vi "HFRR ADV v036.vi"() -> ()   [LabVIEW 2025] (continued)
                    tunnel: w3951 -> [_ _ _ _ _ _ _ _ _ _ _ _ _ _ _]
                    frame 0 {
                      "TITTLE" <- w3958
                    }
                    frame 1 {
                      "Sample ID" <- w3959
                    }
                    frame 2 {
                    }
                    frame 3 {
                    }
                    frame 4 {
                      "Test Date" <- w3960
                    }
                    frame 5 {
                      "Tested by" <- w3961
                    }
                    frame 6 {
                      n2894 = Fract/Exp String To Number(string=w3962) -> (number=→"Humidity before test 2":dbl)  [unwired: 3 in, 1 out]
                    }
                    frame 7 {
                      n2895 = Fract/Exp String To Number(string=w3964) -> (number=→"Temperature before test 2":dbl)  [unwired: 3 in, 1 out]
                    }
                    frame 8 {
                      n2896 = Fract/Exp String To Number(string=w3966) -> (number=→"Humidity after test 2":dbl)  [unwired: 3 in, 1 out]
                    }
                    frame 9 {
                      n2897 = Fract/Exp String To Number(string=w3968) -> (number=→"Temperature after test 2":dbl)  [unwired: 3 in, 1 out]
                    }
                    frame 10 {
                      n2898 = Fract/Exp String To Number(string=w3970) -> (number=→"MWSD 2":dbl)  [unwired: 3 in, 1 out]
                    }
                    frame 11 {
                      n2899 = Fract/Exp String To Number(string=w3972) -> (number=→"AVP 2":dbl)  [unwired: 3 in, 1 out]
                    }
                    frame 12 {
                      n2900 = Fract/Exp String To Number(string=w3974) -> (number=→"HCF 2":dbl)  [unwired: 3 in, 1 out]
                    }
                    frame 13 {
                      n2901 = Fract/Exp String To Number(string=w3976) -> (number=→"WS1.4 2":dbl)  [unwired: 3 in, 1 out]
                    }
                    frame 14, Default {
                    }
                  }
                }
              }
              frame #2 {
              }
            }
            n2902 = local write "OK Button 16"(FALSE ("OK Button 13")) -> ()
          }
        }
        n2903 = Index Array(array=w3621, index="Select Printer 3") -> (element=w3623:string)
        "Selected Printer" <- w3623
        n2904 = case shown="True" w3618 {
          frame False {
          }
          frame True {
            n2905 = flat-sequence {
              frame #0 {
              }
              frame #1 {
                n2906 = Wait (ms)(milliseconds to wait=u32 100) -> ()  [unwired: 1 out]
              }
              frame #2 {
                n2907 = local write "OK Button 16"(FALSE ("Print 3")) -> ()
              }
            }
          }
        }
        n2908 = case shown="True" "Print" {
          tunnel: w3623 -> [_ w3915]
          frame False {
          }
          frame True {
            (unwired) i16 6 ("width (-)")
            (unwired) "TESTED BY : "
            (unwired) "TESTED DATE :"
            (unwired) "SAMPLE ID : "
            (unwired) "SAMPLE DESIGN : "
            w3873 = "\r"
            w3890 = "\r"
            # "add image"
            n2909 = local read "Sample ID"() -> (w3863:string)
            n2910 = local read "Tested by"() -> (w3866:string)
            n2911 = local read "String 34"() -> (w3853:string)
            n2912 = local read "String 45"() -> (w3833:string)
            n2913 = local read "String 35"() -> (w3848:string)
            n2914 = local read "String 37"() -> (w3846:string)
            n2915 = local read "String 32"() -> (w3868:string)
            n2916 = local read "String 36"() -> (w3843:string)
            n2917 = local read "String 31"() -> (w3867:string)
            n2918 = local read "Test Date"() -> (w3864:string)
            n2919 = local read "String 33"() -> (w3869:string)
            n2920 = local read "String 38"() -> (w3839:string)
            n2921 = local read "String 39"() -> (w3836:string)
            n2922 = local write "Print"(FALSE ("Print FF")) -> ()
            n2923 = local read "S 39"() -> (w3851:string)
            n2924 = local read "S 38"() -> (w3858:string)
            n2925 = local read "Temperature before test 2"() -> (w3889:dbl)
            n2926 = local read "Temperature after test 2"() -> (w3879:dbl)
            n2927 = local read "Humidity before test 2"() -> (w3904:dbl)
            n2928 = local read "Humidity after test 2"() -> (w3888:dbl)
            n2929 = local read "MWSD 2"() -> (w3893:dbl)
            n2930 = local read "WS1.4 2"() -> (w3871:dbl)
            n2931 = Concatenate Strings("2)" ("string"), w3853) -> (w3854:string)
            n2932 = Concatenate Strings("3)" ("string"), w3851) -> (w3852:string)
            n2933 = Concatenate Strings("1)" ("string"), w3858) -> (w3857:string)
            n2934 = Concatenate Strings("4)" ("string"), w3848) -> (w3849:string)
            n2935 = Concatenate Strings("5)" ("string"), w3846) -> (w3845:string)
            n2936 = Concatenate Strings("6)" ("string"), w3843) -> (w3842:string)
            n2937 = Concatenate Strings("7)" ("string"), w3839) -> (w3840:string)
            n2938 = Concatenate Strings("8)" ("string"), w3836) -> (w3837:string)
            n2939 = local read "HCF 2"() -> (w3875:dbl)
            n2940 = local read "AVP 2"() -> (w3892:dbl)
            n2941 = local read "s.NO"() -> (w3834:string)
            n2942 = call <vilib>:"New Report.vi"("report type"=enum16{"Standard Report", "HTML"}."Standard Report") -> ("report out"=w3913:refnum<class "NI_report.lvclass">, "error out"=w3912:errorcluster)  [unwired: 13 in]
            n2943 = local read "TITTLE"() -> (w3865:string)
            n2944 = Concatenate Strings(w3890, w3833, w3834, w3890, w3868, w3863, w3890, w3867, w3864, w3890, w3869, w3866, w3890) -> (w3883:string)
            "test by" <- w3883
            n2945 = Number To Fractional String(number=w3889, width (-)=i16 6, precision (6)=i16 2) -> (F-format string=w3878:string)  [unwired: 1 in]
            n2946 = Number To Fractional String(number=w3888, width (-)=i16 6, precision (6)=i16 2) -> (F-format string=w3891:string)  [unwired: 1 in]
            n2947 = Number To Fractional String(number=w3904, width (-)=i16 6, precision (6)=i16 2) -> (F-format string=w3909:string)  [unwired: 1 in]
            n2948 = Number To Fractional String(number=w3893, width (-)=i16 6, precision (6)=i16 2) -> (F-format string=w3895:string)  [unwired: 1 in]
            n2949 = Number To Fractional String(number=w3879, width (-)=i16 6, precision (6)=i16 2) -> (F-format string=w3880:string)  [unwired: 1 in]
            n2950 = Number To Fractional String(number=w3892, width (-)=i16 6, precision (6)=i16 2) -> (F-format string=w3894:string)  [unwired: 1 in]
            n2951 = Number To Fractional String(number=w3875, width (-)=i16 6, precision (6)=i16 2) -> (F-format string=w3874:string)  [unwired: 1 in]
            n2952 = Number To Fractional String(number=w3871, precision (6)=i16 2) -> (F-format string=w3870:string)  [unwired: 2 in]
            n2953 = call-dynamic "Set Report Header Text.vi"("report in"=w3913, "center header text"=w3865, "error in (no error)"=w3912) -> ("report out"=w3884:refnum<class "NI_report.lvclass">, "error out"=w3885:errorcluster)  [unwired: 11 in]
            n2954 = Concatenate Strings(w3873, w3857, w3909, w3873, w3854, w3878, w3873, w3852, w3891, w3873, w3849, w3880, w3873, w3845, w3895, w3873, w3842, w3894, w3873, w3840, w3874, w3873, w3837, w3870) -> (w3861:string)
            "export 2" <- w3861
            n2955 = call-poly <vilib>:"Append Report Text.vi"("report in"=w3884, "text"=w3883, "error in (no error)"=w3885) -> ("report out"=w3887:refnum<class "NI_report.lvclass">, "error out"=w3886:errorcluster)  [unwired: 9 in, 2 out]
            n2956 = local read "test by"() -> (w3860:string)
            n2957 = local read "TITTLE"() -> (w3862:string)
            n2958 = call-poly <vilib>:"Append Report Text.vi"("report in"=w3887, "error in (no error)"=w3886) -> ("report out"=w3908:refnum<class "NI_report.lvclass">, "error out"=w3906:errorcluster)  [unwired: 10 in, 2 out]
            n2959 = Concatenate Strings(w3862, w3861, w3860) -> (→"output":string)
            n2960 = call-poly <vilib>:"Append Report Text.vi"("report in"=w3908, "text"=w3861, "error in (no error)"=w3906) -> ("report out"=w3907:refnum<class "NI_report.lvclass">, "error out"=w3905:errorcluster)  [unwired: 9 in, 2 out]
            n2961 = call-dynamic "Print Report.vi"("report in"=w3907, "printer name (default)"=w3915, "error in (no error)"=w3905) -> ("report out"=w3917:refnum<class "NI_report.lvclass">, "error out"=w3918:errorcluster)  [unwired: 11 in]
            n2962 = call-dynamic "Dispose Report.vi"("report in"=w3917, "error in (no error)"=w3918) -> ()  [unwired: 13 in, 1 out]
          }
        }
        n2963 = case shown="True" "Print 2" {
          frame False {
          }
          frame True {
            n2964 = flat-sequence {
              frame #0 {
                n2965 = local read "s.NO"() -> (→"s.NO 2":string)
                n2966 = Wait (ms)(milliseconds to wait=u32 20) -> ()  [unwired: 1 out]
                n2967 = local read "Sample ID  3"() -> (→"Sample ID  6":string)
                n2968 = local read "Sample ID  4"() -> (→"Sample ID  7":string)
                n2969 = local read "Sample ID"() -> (→"Sample ID  2":string)
                n2970 = local read "Tested by"() -> (→"Tested by 2":string)
                n2971 = local read "Test Date"() -> (→"Test Date 2":string)
                n2972 = local read "Humidity after test 3"() -> (→"Humidity after test 4":dbl)
                n2973 = local read "Ref A Test Date :"() -> (→"TITTLE 4":string)
                n2974 = local read "Temperature before test 3"() -> (w3740:dbl)
                n2975 = local read "Temperature before test 3"() -> (→"Temperature after test 5":dbl)
                n2976 = local read "Temperature after test 3"() -> (→"Temperature after test 4":dbl)
                n2977 = local read "Humidity before test 3"() -> (→"Humidity before test 4":dbl)
                n2978 = local write "Temperature before test 3"(w3740) -> ()
                n2979 = local read "image data"() -> (w3731:T16)
                n2980 = String To Path(string="C:\\LAB-IQ\\im\\Temp_resized.jpg") -> (path=w3732:path)
                "path 2" <- w3732
                n2981 = call <vilib>:"Write JPEG File.vi"("image data"=w3731, "path to JPEG file"=w3732) -> ()  [unwired: 8 in, 2 out]
                "Ref A Test Date :" <- "Ref A Test Date :"
                "Ref B Test Date :" <- "Ref B Test Date :"
                "Ref B Scar Value :" <- "Ref B Scar Value :"
                "Ref A Scar Value :" <- "Ref A Scar Value :"
              }
              frame #1 {
                (unwired) HTML_Report_Image_Alignment."MIDDLE" ("alignment (default)")
                w3768 = u16 0 items=["portrait", "landscape"] ("orientation (portrait)")
                (unwired) HTML_Report_Image_Alignment."ABSMIDDLE" ("alignment (default)")
                (unwired) "TESTED BY : "
                (unwired) "TESTED DATE :"
                (unwired) "SAMPLE ID : "
                (unwired) "SAMPLE DESIGN : "
                w3801 = "\r"
                # "add image"
                n2982 = Wait (ms)(milliseconds to wait=u32 20) -> ()  [unwired: 1 out]
                n2983 = local read "Sample ID  2"() -> (w3794:string)
                n2984 = local read "Wear Scar X"() -> (w3766:dbl)
                "Length ( microns ) 2" <- w3766
                n2985 = local read "Wear Scar Y"() -> (w3765:dbl)
                "Wear Scar Y ( microns ) :" <- w3765
                n2986 = local read "Test Date 2"() -> (w3795:string)
                n2987 = local read "Tested by 2"() -> (w3796:string)
                n2988 = local read "String 46"() -> (w3792:string)
                n2989 = local read "String 48"() -> (w3798:string)
                n2990 = local read "String 47"() -> (w3797:string)
                n2991 = local read "String 49"() -> (w3799:string)
                n2992 = local read "String 10"() -> (w3752:string)
                n2993 = local read "s.NO 2"() -> (w3793:string)
                n2994 = Add(x=w3766, y=w3765) -> (x+y=w3764:dbl)
                n2995 = call <vilib>:"New Report.vi"("report type"=enum16{"Standard Report", "HTML"}."HTML") -> ("report out"=w3772:refnum<class "NI_report.lvclass">, "error out"=w3770:errorcluster)  [unwired: 13 in]
                n2996 = Concatenate Strings(w3801, w3792, w3793, w3801, w3798, w3794, w3801, w3797, w3795, w3801, w3799, w3796, w3801) -> (→"test by 2":string)
                n2997 = Concatenate Strings("C:\\LAB-IQ\\Data\\" ("string"), w3752, ".jpg" ("string")) -> ()  [unwired: 1 out]
                n2998 = Divide(x=w3764, y=2.0) -> (x/y=→"Mean Wear ( microns) :":dbl)
                n2999 = call-dynamic "Set Report Orientation.vi"("report in"=w3772, "orientation (portrait)"=w3768, "error in (no error)"=w3770) -> ("report out"=w3771:refnum<class "NI_report.lvclass">, "error out"=w3769:errorcluster)  [unwired: 11 in]
                n3000 = for {
                  N: 5 -> [_]
                  tunnel: w3771 -> [w3822]
                  tunnel: [w3821] -> w3750
                  tunnel: w3769 -> [w3820]
                  tunnel: [w3819] -> w3749
                  n3001 = call-dynamic "Set Report Tab Width.vi"("report in"=w3822, "error in (no error)"=w3820) -> ("report out"=w3821:refnum<class "NI_report.lvclass">, "error out"=w3819:errorcluster)  [unwired: 12 in]
                }
                n3002 = local read "TITTLE"() -> (w3767:string)
                n3003 = call-dynamic "Set Report Header Text.vi"("report in"=w3750, "center header text"=w3767, "error in (no error)"=w3749) -> ("report out"=w3788:refnum<class "NI_report.lvclass">, "error out"=w3787:errorcluster)  [unwired: 11 in]
                n3004 = for {
                  N: 1 -> [_]
                  tunnel: [w3826] -> w3774
                  tunnel: [w3825] -> w3773
                  tunnel: w3788 -> [w3824]
                  tunnel: w3787 -> [w3823]
                  n3005 = call-dynamic "New Report Line.vi"("report in"=w3824, "error in (no error)"=w3823) -> ("report out"=w3826:refnum<class "NI_report.lvclass">, "error out"=w3825:errorcluster)  [unwired: 12 in]
                }
                n3006 = for {
                  N: 2 -> [_]
                  tunnel: [w3818] -> w3780
                  tunnel: [w3817] -> w3779
                  tunnel: w3774 -> [w3816]
                  tunnel: w3773 -> [w3815]
                  n3007 = call-dynamic "New Report Line.vi"("report in"=w3816, "error in (no error)"=w3815) -> ("report out"=w3818:refnum<class "NI_report.lvclass">, "error out"=w3817:errorcluster)  [unwired: 12 in]
                }
                n3008 = for {
                  N: 25 -> [_]
                  tunnel: w3780 -> [w3814]
                  tunnel: w3779 -> [w3812]
                  tunnel: [w3813] -> w3783
                  tunnel: [w3811] -> w3782
                  n3009 = call-dynamic "Set Report Tab Width.vi"("report in"=w3814, "error in (no error)"=w3812) -> ("report out"=w3813:refnum<class "NI_report.lvclass">, "error out"=w3811:errorcluster)  [unwired: 12 in]
                }
                n3010 = control-ref of="Tab Control 9"() -> (w3778:refnum<vi>)
                n3011 = call-dynamic "Append Control Image to Report.vi"("report in"=w3783, "alignment (default)"=HTML_Report_Image_Alignment."ABSMIDDLE", "ctrl reference"=w3778, "error in (no error)"=w3782) -> ("report out"=w3777:refnum<class "NI_report.lvclass">, "error out"=w3776:errorcluster)  [unwired: 8 in, 2 out]
                n3012 = for {
                  N: 3 -> [_]
                  tunnel: [w3810] -> w3761
                  tunnel: [w3809] -> w3760
                  tunnel: w3777 -> [w3808]
                  tunnel: w3776 -> [w3807]
                  n3013 = call-dynamic "New Report Line.vi"("report in"=w3808, "error in (no error)"=w3807) -> ("report out"=w3810:refnum<class "NI_report.lvclass">, "error out"=w3809:errorcluster)  [unwired: 12 in]
                }
                n3014 = for {
                  N: 100 -> [_]
                  tunnel: w3761 -> [w3806]
                  tunnel: w3760 -> [w3804]
                  tunnel: [w3805] -> w3757
                  tunnel: [w3803] -> w3755
                  n3015 = call-dynamic "Set Report Tab Width.vi"("report in"=w3806, "error in (no error)"=w3804) -> ("report out"=w3805:refnum<class "NI_report.lvclass">, "error out"=w3803:errorcluster)  [unwired: 12 in]
                }
                n3016 = String To Path(string="C:\\LAB-IQ\\im\\Temp_resized.jpg") -> (path=w3747:path)
                n3017 = call-poly <vilib>:"Append Image to Report.vi"("report in"=w3757, "path or URL of image"=w3747, "error in (no error)"=w3755) -> ("report out"=w3756:refnum<class "NI_report.lvclass">, "error out"=w3754:errorcluster)  [unwired: 9 in, 2 out]
                n3018 = call-poly <vilib>:"Open HTML Report in Browser.vi"("report in"=w3756, "error in (no error)"=w3754) -> ("report out"=w3791:refnum<class "NI_report.lvclass">, "error out"=w3790:errorcluster)  [unwired: 11 in, 1 out]
                n3019 = call-dynamic "Dispose Report.vi"("report in"=w3791, "error in (no error)"=w3790) -> ()  [unwired: 13 in, 1 out]
              }
              frame #2 {
              }
              frame #3 {
                n3020 = disable-structure shown="Disabled" {
                  frame Disabled {
                    n3021 = local read "String 10"() -> (w3831:string)
                    n3022 = Concatenate Strings("C:\\LAB-IQ-NXT\\Data\\" ("string"), w3831, ".jpg" ("string")) -> (w3829:string)
                    n3023 = String To Path(string=w3829) -> (path=w3828:path)
                    n3024 = Delete(path (use dialog)=w3828) -> ()  [unwired: 4 in, 3 out]
                  }
                  frame Enabled {
                  }
                }
                n3025 = local write "Print 2"(FALSE ("Print")) -> ()
              }
            }
          }
        }
      }
    }
    n3026 = Wait (ms)(milliseconds to wait=u32 50) -> ()  [unwired: 1 out]
    n3027 = Wait (ms)(milliseconds to wait=u32 50) -> ()  [unwired: 1 out]
    n3028 = local read "Quit"() -> (w2175:bool)
  }
  n3029 = VISA Close(VISA resource name=w41, error in (no error)=w40) -> ()  [unwired: 1 out]
  n3030 = while {
    stop <- w3982 stop-if-true
    n3031 = local read "Auto Start Test"() -> (w3980:bool)
    n3032 = local read "RUN"() -> (w3979:bool)
    n3033 = Wait (ms)(milliseconds to wait=u32 1000) -> ()  [unwired: 1 out]
    n3034 = Or(x=w3979, y=w3980) -> (x .or. y?=w3978:bool)
    n3035 = case shown="True" w3978 {
      frame False {
      }
      frame True {
        n3036 = local read "LVDT STROKE Actual"() -> (w3983:dbl)
        n3037 = In Range and Coerce(upper limit=1.2, x=w3983, lower limit=0.6) -> (In Range?=w3986:bool)  [unwired: 1 out]
        n3038 = call-poly <vilib>:"Random Number (Range).vi"("lower bound (0)"=0.998 ("upper bound (100)"), "upper bound (100)"=1.003) -> ("number"=w3984:dbl)  [unwired: 9 in]
        n3039 = case shown="True" w3986 {
          tunnel: [w3991 w3992] -> w3985
          tunnel: w3984 -> [_ w3992]
          tunnel: w3983 -> [w3991 _]
          frame False {
          }
          frame True {
          }
        }
        "LVDT STROKE DISPLAY" <- w3985
      }
    }
    n3040 = local read "Quit"() -> (w3982:bool)
  }
  n3041 = while {
    tunnel: [w4009] -> w49
    shift-right: [w4002] -> _
    shift-left: 0.0 -> [w4005]
    shift-right: [w4001] -> _
    shift-left: 0.0 -> [w4004]
    shift-right: [w4000] -> _
    shift-left: 100.0 ("vc_cmd") -> [w4003]
    stop <- w4009 stop-if-true
    # "PID LOGIC"
    n3042 = local read "run test Calibration"() -> (w3997:bool)
    n3043 = local read "RUN"() -> (w4007:bool)
    n3044 = local read "Auto Start Temp"() -> (w3998:bool)
    n3045 = local read "Auto Start Test"() -> (w4006:bool)
    n3046 = local read "START TEMP"() -> (w3996:bool)
    n3047 = And(x=w3998, y=w4006) -> (x .and. y?=w3999:bool)
    n3048 = Or(x=w4007, y=w3999) -> (x .or. y?=w4008:bool)
    n3049 = And(x=w4008, y=w3996) -> (x .and. y?=w3995:bool)
    n3050 = And(x=w3997, y=w3996) -> (x .and. y?=w3994:bool)
    n3051 = Or(x=w3994, y=w3995) -> (x .or. y?=w3993:bool)
    n3052 = Wait (ms)(milliseconds to wait="milliseconds to wait") -> ()  [unwired: 1 out]
    n3053 = case shown="True" w3993 {
      tunnel: [400.0 ("out_vc_cmd") w4028] -> w4000
      tunnel: [w4012 w4030] -> w4001
      tunnel: [w4012 w4029] -> w4002
      tunnel: w4005 -> [_ w4019]
      tunnel: w4004 -> [_ w4018]
      tunnel: w4003 -> [_ w4017]
      tunnel: w3997 -> [_ w4013]
      frame False {
        w4012 = 0.0 ("error_out")
      }
      frame True {
        n3054 = case shown="True" w4013 {
          tunnel: [w4037 1.0] -> w4015
          frame False {
            n3055 = local read "Set Strk"() -> (w4036:dbl)
            n3056 = Add(x=w4036, y="Add up Stroke") -> (x+y=w4037:dbl)
          }
          frame True {
          }
        }
        n3057 = local read "LVDT STROKE"() -> (w4014:dbl)
        n3058 = formula code="// Zero-Hardcode Explicit Positional-Form PID Engine\n// Inputs: target_stroke, measured_stroke, dt, prev_error, integral_accumulator_in, prev_vc_cmd\n//         kp, ki, kd, max_step_change, max_amplitude, min_amplitude, startup_cmd\n// Outputs: vc_cmd, error_out, out_error, integral_accumulator_out, out_vc_cmd\n\n// 1. Calculate Tracking Error\nfloat current_error = target_stroke - measured_stroke;\nerror_out = current_error;\n\n// 2. Compute Proportional Term\nfloat p_term = kp * current_error;\n\n// 3. Compute Derivative Term\nfloat d_term = 0.0;\nif (dt > 0.0) {\n    d_term = kd * ((current_error - prev_error) / dt);\n}\n\n// 4. Update and Accumulate Integral Term\nfloat current_integral = integral_accumulator_in + (current_error * dt);\nfloat i_term = ki * current_integral;\n\n// 5. Calculate Ideal Target Command (Anchored by startup baseline)\nfloat ideal_command = startup_cmd + p_term + i_term + d_term;\n\n// 6. Apply Loop Rate Limiting FIRST \n// (Forces the command to climb gradually from prev_vc_cmd instead of jumping straight to max)\nfloat raw_adjustment = ideal_command - prev_vc_cmd;\n\nif (raw_adjustment > max_step_change) {\n    raw_adjustment = max_step_change;\n} else if (raw_adjustment < -max_step_change) {\n    raw_adjustment = -max_step_change;\n}\n\nfloat next_vc_cmd = prev_vc_cmd + raw_adjustment;\n\n// 7. Anti-Windup Protection & Final Output Safety Safeguard Clamping\n// (Back-calculating based on what we are ACTUALLY outputting)\nif (next_vc_cmd > max_amplitude) {\n    float excess = next_vc_cmd - max_amplitude;\n    if (ki > 0.0) {\n        current_integral -= excess / ki;\n    }\n    next_vc_cmd = max_amplitude;\n} else if (next_vc_cmd < min_amplitude) {\n    float excess = next_vc_cmd - min_amplitude;\n    if (ki > 0.0) {\n        current_integral -= excess / ki;\n    }\n    next_vc_cmd = min_amplitude;\n}\n\n// 8. Map to Shift Registers for memory persistence\nvc_cmd = next_vc_cmd;\nout_error = current_error;                   \nintegral_accumulator_out = current_integral;  \nout_vc_cmd = next_vc_cmd;"("target_stroke"=w4015, "measured_stroke"=w4014, "dt"="dt", "integral_accumulator_in"=w4018, "prev_error"=w4019, "prev_vc_cmd"=w4017, "kp"="kp", "ki"="ki", "kd"="kd", "max_step_change"="max_step_change", "max_amplitude"="max_amplitude", "min_amplitude"="min_amplitude", "startup_cmd"="startup_cmd") -> ("vc_cmd"=w4034:dbl, "out_error"=w4029:dbl, "integral_accumulator_out"=w4030:dbl, "out_vc_cmd"=w4028:dbl)  [unwired: 1 out]
        "output Vpp" <- w4034
        n3059 = Number To Fractional String(number=w4034, precision (6)=i16 1) -> (F-format string=w4032:string)  [unwired: 2 in]
        n3060 = Concatenate Strings("DAC;" ("string"), w4032) -> (w4016:string)
        n3061 = local write "Due Write"(w4016) -> ()
        "prev_error" <- w4019
        "integral_accumulator_in" <- w4018
        "prev_vc_cmd" <- w4017
      }
    }
    n3062 = local read "Quit"() -> (w4009:bool)
  }
  n3063 = Or(x=w45, y=w44) -> (x .or. y?=w46:bool)
  n3064 = Or(x=w42, y=w46) -> (x .or. y?=w51:bool)
  n3065 = control-ref of="new picture"() -> ()  [unwired: 1 out]
  n3066 = Or(x=w54, y=w51) -> (x .or. y?=w48:bool)
  n3067 = Or(x=w48, y=w49) -> (x .or. y?=w43:bool)
  n3068 = while {
    tunnel: [w4039] -> w53
    i -> [w4046]
    stop <- w4039 stop-if-true
    n3069 = local read "Quit"() -> (w4039:bool)
    n3070 = Equal To 0?(x=w4046) -> (x = 0?=w4044:bool)
    n3071 = call "Elapsed Time3"("Time Target (s)"=45.0, "Auto Reset"=TRUE) -> ("Time has Elapsed"=w4043:bool)  [unwired: 10 in, 7 out]
    n3072 = Wait (ms)(milliseconds to wait=u32 50) -> ()  [unwired: 1 out]
    n3073 = Or(x=w4043, y=w4044) -> (x .or. y?=w4045:bool)
    n3074 = case shown="True" w4045 {
      frame False {
      }
      frame True {
        n3075 = call <vilib>:"System Exec.vi"("run minimized? (F)"=TRUE, "error in (no error)"="error in (no error)", "command line"="powercfg.exe -change -monitor-timeout-ac 0") -> ("error out"=w4057:errorcluster)  [unwired: 5 in, 3 out]
        n3076 = call <vilib>:"System Exec.vi"("run minimized? (F)"=TRUE, "error in (no error)"=w4057, "command line"="powercfg.exe -change -disk-timeout-ac 0") -> ("error out"=w4056:errorcluster)  [unwired: 5 in, 3 out]
        n3077 = call <vilib>:"System Exec.vi"("run minimized? (F)"=TRUE, "error in (no error)"=w4056, "command line"="powercfg.exe -change -standby-timeout-ac 0") -> ("error out"=w4055:errorcluster)  [unwired: 5 in, 3 out]
        n3078 = call <vilib>:"System Exec.vi"("run minimized? (F)"=TRUE, "error in (no error)"=w4055, "command line"="powercfg.exe -change -hibernate-timeout-ac 0") -> ("error out"=w4054:errorcluster)  [unwired: 5 in, 3 out]
        n3079 = call <vilib>:"Simple Error Handler.vi"("error in (no error)"=w4054) -> ("error out"=w4060:errorcluster)  [unwired: 4 in, 4 out]
        n3080 = call <vilib>:"Clear Errors.vi"("error in (no error)"=w4060) -> ("error out"=→"error out":errorcluster)  [unwired: 5 in, 1 out]
      }
    }
  }
  n3081 = Compound Arithmetic op=OR(w56, w43, w53) -> (w55:bool)
  n3082 = flat-sequence {
    tunnel: w55 -> [_]
    tunnel: [w4062] -> w25
    tunnel: w25 -> [_]
    frame #0 {
      n3083 = call "CLOSE CONNECTION.vi"() -> ("error out"=w4062:errorcluster)  [unwired: 11 in]
    }
    frame #1 {
      n3084 = Quit LabVIEW(quit? (T)=TRUE) -> ()
      n3085 = local write "Quit"(FALSE ("EXIT")) -> ()
    }
  }
  n3086 = property on="Heater Button" class="Bool (strict)"("Visible"=TRUE) -> ()  [unwired: 2 in, 2 out]
  n3087 = while {
    tunnel: [w4069] -> _
    i -> [w4069]
    stop <- w4065 stop-if-true
    # "Langauage selection"
    n3088 = Equal?(x="Lan flag", y=22.0) -> ()  [unwired: 1 out]
    n3089 = disable-structure shown="Disabled" {
      frame Disabled {
        n3090 = stacked-sequence {
          frame #0 {
            n3091 = case shown="\"Russian\"" "Language Selection" {
              tunnel: [0 1] -> w4071
              frame "English", Default {
              }
              frame "Russian" {
              }
            }
            n3092 = for {
              N: 130 -> [_]
              tunnel: "Table" -> [w4080]
              tunnel: w4071 -> [w4079]
              i -> [w4078]
              n3093 = Index Array(array=w4080, index (row)=w4078, index (col)=w4079) -> (element=w4077:string)
              n3094 = case shown="1" w4078 {
                tunnel: w4077 -> [w4081 w4082 _ w4083 w4084 w4085 w4086 w4087 w4088 w4089 w4090 w4091 w4092 w4093 w4094 w4095 w4096 w4097 w4098 w4099 w4100 w4101 w4102 w4103 w4104 w4105 w4106 w4107 w4108 _ _ w4109 w4110 w4111 w4112 w4113 w4114 w4123 w4130 w4137 w4144 w4148 w4151 w4154 w4156 w4158 w4159 w4160 w4161 w4162 w4163 w4164 w4165 w4166 w4167 w4168 w4169 w4170 w4171 w4172 w4173 w4174 w4175 w4176 w4177 w4178 w4179 w4180 w4181 w4182 w4183 w4184 w4185 w4186 w4187 w4188 w4189 w4190 w4191 w4192 w4193 w4194 w4195 w4196 w4197 w4198 w4199 w4200 w4201 w4202 w4203 w4204 w4205 w4206 w4207 w4208 w4209 w4210 w4211 w4212 w4213 w4214 w4215 w4216 w4217 _ w4218 w4219 w4220 w4221 w4222 w4223 w4224 w4225 w4226 w4227 w4228 w4229 w4230 _ w4231 w4232 w4233 w4234 w4235 w4236 _]
                frame 0 {
                  n3095 = local write "S"(w4081) -> ()
                }
                frame 1 {
                  n3096 = local write "S 2"(w4082) -> ()
                }
                frame 2 {
                }
                frame 3 {
                  n3097 = local write "S 4"(w4083) -> ()
                }
                frame 4 {
                  n3098 = property on="FILE" class="Str"("Caption.Text"=w4084) -> ()  [unwired: 2 in, 2 out]
                }
                frame 5 {
                  n3099 = property on="Fuel Discription :" class="Str"("Caption.Text"=w4085) -> ()  [unwired: 2 in, 2 out]
                }
                frame 6 {
                  n3100 = property on="Remarks :" class="Str"("Caption.Text"=w4086) -> ()  [unwired: 2 in, 2 out]
                }
                frame 7 {
                  n3101 = property on="Save & Continue" class="Bool (strict)"("Boolean Text.Text"=w4087) -> ()  [unwired: 2 in, 2 out]
                }
                frame 8 {
                }
                frame 9 {
                  n3102 = property on="Set Hz" class="DigNum (strict)"("Caption.Text"=w4089) -> ()  [unwired: 2 in, 2 out]
                }
                frame 10 {
                }
                frame 11 {
                  n3103 = property on="NORMAL LOAD" class="DigNum (strict)"("Caption.Text"=w4091) -> ()  [unwired: 2 in, 2 out]
                }
                frame 12 {
                }
                frame 13 {
                  n3104 = property on="Set Temp" class="DigNum (strict)"("Caption.Text"=w4093) -> ()  [unwired: 2 in, 2 out]
                }
                frame 14 {
                  n3105 = local write "S 15"(w4094) -> ()
                }
                frame 15 {
                  n3106 = property on="Set Rh" class="DigNum (strict)"("Caption.Text"=w4095) -> ()  [unwired: 2 in, 2 out]
                }
                frame 16 {
                }
                frame 17 {
                  n3107 = local write "S 18"(w4097) -> ()
                }
                frame 18 {
                  "String 17" <- w4098
                }
                frame 19 {
                  n3108 = property on="test time" class="DigNum (strict)"("Caption.Text"=w4099) -> ()  [unwired: 2 in, 2 out]
                }
                frame 20 {
                  "String 18" <- w4100
                  "String 22" <- w4100
                }
                frame 21 {
                  n3109 = property on="Elapsed time" class="DigNum (strict)"("Caption.Text"=w4101) -> ()  [unwired: 2 in, 2 out]
                }
                frame 22 {
                  n3110 = property on="Samplingtime 2" class="DigNum (strict)"("Caption.Text"=w4102) -> ()  [unwired: 2 in, 2 out]
                }
                frame 23 {
                  "String 21" <- w4103
                }
                frame 24 {
                  n3111 = property on="Countdown" class="DigNum (strict)"("Caption.Text"=w4104) -> ()  [unwired: 2 in, 2 out]
                }
                frame 25 {
                  n3112 = property on="Countdown 2" class="DigNum (strict)"("Caption.Text"=w4105) -> ()  [unwired: 2 in, 2 out]
                }
                frame 26 {
                  n3113 = property on="Engage" class="Bool (strict)"("Boolean Text.Text"=w4106) -> ()  [unwired: 2 in, 2 out]
                }
                frame 27 {
                  n3114 = property on="Boolean  4" class="Bool (strict)"("Boolean Text.Text"=w4107) -> ()  [unwired: 2 in, 2 out]
                }
                frame 28 {
                  n3115 = property on="Test \nStatus" class="Bool (strict)"("Boolean Text.Text"=w4108) -> ()  [unwired: 2 in, 2 out]
                }
                frame 29 {
                }
                frame 30 {
                }
                frame 31 {
                }
                frame 32 {
                  n3116 = property on="RSTCOF" class="Bool"("Boolean Text.Text"=w4110) -> ()  [unwired: 2 in, 2 out]
                  n3117 = property on="RST FF" class="Bool"("Boolean Text.Text"=w4110) -> ()  [unwired: 2 in, 2 out]
                  n3118 = property on="RST TEMP" class="Bool"("Boolean Text.Text"=w4110) -> ()  [unwired: 2 in, 2 out]
                  n3119 = property on="RSTV1 3" class="Bool"("Boolean Text.Text"=w4110) -> ()  [unwired: 2 in, 2 out]
                  n3120 = property on="rstv2" class="Bool"("Boolean Text.Text"=w4110) -> ()  [unwired: 2 in, 2 out]
                  n3121 = property on="RSTV1 2" class="Bool"("Boolean Text.Text"=w4110) -> ()  [unwired: 2 in, 2 out]
                  n3122 = property on="RST CP" class="Bool"("Boolean Text.Text"=w4110) -> ()  [unwired: 2 in, 2 out]
                }
                frame 33 {
                  "S 61" <- w4111
                }
                frame 34 {
                  "String 23" <- w4112
                }
                frame 35 {
                  n3123 = property on="Rh Before" class="DigNum (strict)"("Caption.Text"=w4113) -> ()  [unwired: 2 in, 2 out]
                }
                frame 36 {
                  n3124 = Match Pattern(string=w4114, regular expression=",") -> (before substring=→"bs":string, after substring=→"as":string)  [unwired: 1 in, 2 out]
                  n3125 = property on="Rh After" class="DigNum (strict)"("Caption.Text"=w4114) -> ()  [unwired: 2 in, 2 out]
                }
                frame 37 {
                  n3126 = Match Pattern(string=w4123, regular expression=",") -> (before substring=w4122:string, after substring=w4121:string)  [unwired: 1 in, 2 out]
                  "bs" <- w4122
                  "as" <- w4121
                  n3127 = Concatenate Strings(w4122, w4121) -> (w4118:string)
                  n3128 = property on="Humidity before test 2" class="DigNum (strict)"("Caption.Text"=w4118) -> ()  [unwired: 2 in, 2 out]
                  n3129 = Concatenate Strings(w4118, "=" ("string")) -> (w4119:string)
                  n3130 = local write "S 38"(w4119) -> ()
                }
                frame 38 {
                  n3131 = Match Pattern(string=w4130, regular expression=",") -> (before substring=w4129:string, after substring=w4128:string)  [unwired: 1 in, 2 out]
                  "bs" <- w4129
                  "as" <- w4128
                  n3132 = Concatenate Strings(w4129, w4128) -> (w4125:string)
                  n3133 = property on="Humidity after test 2" class="DigNum (strict)"("Caption.Text"=w4125) -> ()  [unwired: 2 in, 2 out]
                  n3134 = Concatenate Strings(w4125, "=" ("string")) -> (w4127:string)
                  n3135 = local write "S 39"(w4127) -> ()
                }
                frame 39 {
                  n3136 = Match Pattern(string=w4137, regular expression=",") -> (before substring=w4136:string, after substring=w4135:string)  [unwired: 1 in, 2 out]
                  "bs" <- w4136
                  "as" <- w4135
                  n3137 = Concatenate Strings(w4136, w4135) -> (w4132:string)
                  n3138 = property on="Temperature before test 2" class="DigNum (strict)"("Caption.Text"=w4132) -> ()  [unwired: 2 in, 2 out]
                  n3139 = Concatenate Strings(w4132, "=" ("string")) -> (→"String 34":string)
                }
                frame 40 {
                  n3140 = Match Pattern(string=w4144, regular expression=",") -> (before substring=w4143:string, after substring=w4142:string)  [unwired: 1 in, 2 out]
                  "bs" <- w4143
                  "as" <- w4142
                  n3141 = Concatenate Strings(w4143, w4142) -> (w4139:string)
                  n3142 = property on="Temperature after test 2" class="DigNum (strict)"("Caption.Text"=w4139) -> ()  [unwired: 2 in, 2 out]
                  n3143 = Concatenate Strings(w4139, "=" ("string")) -> (→"String 35":string)
                  n3144 = property on="Temperature after test" class="DigNum (strict)"("Caption.Text"=w4139) -> ()  [unwired: 2 in, 2 out]
                }
                frame 41 {
                  n3145 = property on="AVP 2" class="DigNum (strict)"("Caption.Text"=w4148) -> ()  [unwired: 2 in, 2 out]
                  n3146 = Concatenate Strings(w4148, "=" ("string")) -> (→"String 36":string)
                }
                frame 42 {
                  n3147 = property on="MWSD 2" class="DigNum (strict)"("Caption.Text"=w4151) -> ()  [unwired: 2 in, 2 out]
                  n3148 = Concatenate Strings(w4151, "=" ("string")) -> (→"String 37":string)
                }
                frame 43 {
                  n3149 = property on="HCF 2" class="DigNum (strict)"("Caption.Text"=w4154) -> ()  [unwired: 2 in, 2 out]
                  n3150 = Concatenate Strings(w4154, "=" ("string")) -> (→"String 38":string)
                }
                frame 44 {
                  n3151 = Concatenate Strings(w4156, "=" ("string")) -> (→"String 39":string)
                  n3152 = property on="WS1.4 2" class="DigNum (strict)"("Caption.Text"=w4156) -> ()  [unwired: 2 in, 2 out]
                }
                frame 45 {
                }
                frame 46 {
                  n3153 = local write "S 47"(w4159) -> ()
                }
                frame 47 {
                  n3154 = local write "S 48"(w4160) -> ()
                }
                frame 48 {
                  n3155 = local write "S 49"(w4161) -> ()
                }
                frame 49 {
                  n3156 = local write "S 50"(w4162) -> ()
                }
                frame 50 {
                  n3157 = local write "S 51"(w4163) -> ()
                }
                frame 51 {
                  n3158 = local write "S 52"(w4164) -> ()
                }
                frame 52 {
                  n3159 = local write "S 53"(w4165) -> ()
                }
                frame 53 {
                  n3160 = local write "S 54"(w4166) -> ()
                }
                frame 54 {
                  n3161 = local write "S 55"(w4167) -> ()
                }
                frame 55 {
                  n3162 = local write "S 56"(w4168) -> ()
                }
                frame 56 {
                  n3163 = local write "S 57"(w4169) -> ()
                }
                frame 57 {
                  n3164 = local write "S 58"(w4170) -> ()
                }
                frame 58 {
                  n3165 = local write "S 59"(w4171) -> ()
                }
                frame 59 {
                  n3166 = local write "S 60"(w4172) -> ()
                }
                frame 60 {
                  n3167 = local write "S 62"(w4173) -> ()
                }
                frame 61 {
                  n3168 = local write "S 63"(w4174) -> ()
                }
                frame 62 {
                  n3169 = local write "S 64"(w4175) -> ()
                }
                frame 63 {
                  n3170 = local write "S 65"(w4176) -> ()
                }
                frame 64 {
                  n3171 = local write "S 66"(w4177) -> ()
                }
                frame 65 {
                  n3172 = local write "S 67"(w4178) -> ()
                }
                frame 66 {
                  n3173 = local write "S 68"(w4179) -> ()
                }
                frame 67 {
                  n3174 = local write "S 69"(w4180) -> ()
                }
                frame 68 {
                  n3175 = local write "S 70"(w4181) -> ()
                }
                frame 69 {
                  n3176 = local write "S 71"(w4182) -> ()
                }
                frame 70 {
                  n3177 = local write "S 72"(w4183) -> ()
                }
                frame 71 {
                  n3178 = local write "S 73"(w4184) -> ()
                }
                frame 72 {
                  n3179 = local write "S 74"(w4185) -> ()
                }
                frame 73 {
                  n3180 = local write "S 75"(w4186) -> ()
                }
                frame 74 {
                  n3181 = local write "S 76"(w4187) -> ()
                }
                frame 75 {
                  n3182 = local write "S 77"(w4188) -> ()
                }
                frame 76 {
                  n3183 = local write "S 78"(w4189) -> ()
                }
                frame 77 {
                  n3184 = local write "S 79"(w4190) -> ()
                }
                frame 79 {
                  n3185 = property on="Sample Temperature ( °C )" class="XYGraph (strict)"("Y Scale.Name Label.Text"=w4191) -> ()  [unwired: 2 in, 2 out]
                }
                frame 80 {
                  n3186 = local write "S 81"(w4192) -> ()
                  n3187 = property on="Humidity ( %RH )" class="XYGraph (strict)"("Y Scale.Name Label.Text"=w4192) -> ()  [unwired: 2 in, 2 out]
                }
                frame 78 {
                  n3188 = property on="Air Temperature  ( °C )" class="XYGraph (strict)"("X Scale.Name Label.Text"=w4193) -> ()  [unwired: 2 in, 2 out]
                  n3189 = property on="Humidity ( %RH )" class="XYGraph (strict)"("X Scale.Name Label.Text"=w4193) -> ()  [unwired: 2 in, 2 out]
                  n3190 = property on="Sample Temperature ( °C )" class="XYGraph (strict)"("X Scale.Name Label.Text"=w4193) -> ()  [unwired: 2 in, 2 out]
                  n3191 = property on="Coefficient Of Friction" class="XYGraph (strict)"("X Scale.Name Label.Text"=w4193) -> ()  [unwired: 2 in, 2 out]
                }
                frame 81 {
                  n3192 = property on="Air Temperature  ( °C )" class="XYGraph (strict)"("Y Scale.Name Label.Text"=w4194) -> ()  [unwired: 2 in, 2 out]
                }
                frame 82 {
                  n3193 = local write "S 84"(w4195) -> ()
                }
                frame 83 {
                  n3194 = local write "S 85"(w4196) -> ()
                }
                frame 84 {
                  n3195 = local write "S 86"(w4197) -> ()
                }
                frame 85 {
                  n3196 = local write "S 87"(w4198) -> ()
                }
                frame 86 {
                  n3197 = local write "S 88"(w4199) -> ()
                }
                frame 87 {
                }
                frame 88 {
                  n3198 = local write "S 90"(w4201) -> ()
                }
                frame 89 {
                  n3199 = local write "S 91"(w4202) -> ()
                }
                frame 90 {
                  n3200 = local write "S 92"(w4203) -> ()
                }
                frame 91 {
                  n3201 = local write "S 93"(w4204) -> ()
                }
                frame 92 {
                  n3202 = local write "S 94"(w4205) -> ()
                }
                frame 93 {
                  n3203 = local write "S 95"(w4206) -> ()
                }
                frame 94 {
                  n3204 = local write "S 96"(w4207) -> ()
                }
                frame 95 {
                  n3205 = local write "S 97"(w4208) -> ()
                }
                frame 96 {
                  n3206 = local write "S 98"(w4209) -> ()
                }
                frame 97 {
                  n3207 = local write "S 99"(w4210) -> ()
                }
                frame 98 {
                  n3208 = local write "S 100"(w4211) -> ()
                }
                frame 99 {
                  n3209 = local write "S 101"(w4212) -> ()
                }
                frame 100 {
                  n3210 = local write "S 102"(w4213) -> ()
                }
                frame 101 {
                  n3211 = local write "S 103"(w4214) -> ()
                }
                frame 102 {
                  n3212 = local write "S 104"(w4215) -> ()
                }
                frame 103 {
                  n3213 = local write "S 105"(w4216) -> ()
                }
                frame 104 {
                  n3214 = local write "S 106"(w4217) -> ()
                }
                frame 105 {
                }
                frame 106 {
                  n3215 = property on="OK Button 17" class="Bool (strict)"("Boolean Text.Text"=w4218) -> ()  [unwired: 2 in, 2 out]
                }
                frame 107 {
                  n3216 = property on="OK Button 16" class="Bool (strict)"("Boolean Text.Text"=w4219) -> ()  [unwired: 2 in, 2 out]
                }
                frame 108 {
                  n3217 = property on="TITTLE" class="Str"("Caption.Text"=w4220) -> ()  [unwired: 2 in, 2 out]
                }
                frame 109 {
                  "String 30" <- w4221
                }
                frame 110 {
                  n3218 = property on="Test Date" class="Str"("Caption.Text"=w4222) -> ()  [unwired: 2 in, 2 out]
                  "String 31" <- w4222
                }
                frame 111 {
                  n3219 = property on="Sample ID" class="Str"("Caption.Text"=w4223) -> ()  [unwired: 2 in, 2 out]
                  "String 32" <- w4223
                }
                frame 112 {
                  n3220 = property on="Tested by" class="Str"("Caption.Text"=w4224) -> ()  [unwired: 2 in, 2 out]
                  "String 33" <- w4224
                }
                frame 113 {
                  n3221 = property on="System Configured Printers 2" class="Arr (strict)"("Caption.Text"=w4225) -> ()  [unwired: 2 in, 2 out]
                }
                frame 114 {
                  n3222 = property on="Selected Printer" class="Str"("Caption.Text"=w4226) -> ()  [unwired: 2 in, 2 out]
                }
                frame 115 {
                  n3223 = property on="Select Printer 3" class="DigNum (strict)"("Caption.Text"=w4227) -> ()  [unwired: 2 in, 2 out]
                }
                frame 116 {
                  n3224 = property on="Print" class="Bool (strict)"("Boolean Text.Text"=w4228) -> ()  [unwired: 2 in, 2 out]
                }
                frame 117 {
                  "String 41" <- w4229
                }
                frame 118 {
                  n3225 = property on="tested by" class="Str"("Caption.Text"=w4230) -> ()  [unwired: 2 in, 2 out]
                }
                frame 119 {
                }
                frame 120 {
                  n3226 = property on="Export" class="Bool (strict)"("Boolean Text.Text"=w4231) -> ()  [unwired: 2 in, 2 out]
                }
                frame 121 {
                }
                frame 122 {
                }
                frame 123 {
                  n3227 = property on="Select File Type" class="Enum (strict)"("Caption.Text"=w4234) -> ()  [unwired: 2 in, 2 out]
                }
                frame 124 {
                  n3228 = property on="s.NO" class="Str"("Caption.Text"=w4235) -> ()  [unwired: 2 in, 2 out]
                  "String 45" <- w4235
                }
                frame 125 {
                  n3229 = property on="trip1 8" class="Bool (strict)"("Boolean Text.Text"=w4236) -> ()  [unwired: 2 in, 2 out]
                }
                frame 126, Default {
                }
              }
            }
          }
          frame #1 {
            w4244 = TRUE ("Visible")
            n3230 = local read "S 91"() -> (w4261:string)
            n3231 = local read "S 90"() -> (w4260:string)
            n3232 = local read "S 88"() -> (w4259:string)
            n3233 = property on="File Path" class="Path"("Caption.Text"=w4260) -> ()  [unwired: 2 in, 2 out]
            n3234 = local read "S 71"() -> (w4254:string)
            n3235 = local read "S 86"() -> (w4256:string)
            n3236 = local read "S 85"() -> (w4257:string)
            n3237 = local read "S 87"() -> (w4255:string)
            n3238 = local read "S 84"() -> (w4258:string)
            n3239 = local read "S 103"() -> (w4243:string)
            n3240 = local read "S 104"() -> (w4242:string)
            n3241 = property on="Password" class="Str"("Caption.Text"=w4257) -> ()  [unwired: 2 in, 2 out]
            n3242 = property on="EDIT" class="Bool (strict)"("Boolean Text.Text"=w4254) -> ()  [unwired: 2 in, 2 out]
            n3243 = property on="SAVE" class="Bool (strict)"("Boolean Text.Text"=w4258) -> ()  [unwired: 2 in, 2 out]
            n3244 = Build Array(w4243, w4242) -> (w4241:string[])
            n3245 = property on="Heater Button" class="Bool (strict)"("Strings [4]"=w4241) -> ()  [unwired: 2 in, 2 out]
            n3246 = local read "S 92"() -> (w4253:string)
            n3247 = local read "S 93"() -> (w4252:string)
            n3248 = local read "S 105"() -> (w4239:string)
            n3249 = local read "S 106"() -> (w4238:string)
            n3250 = Build Array(w4253, w4252) -> ()  [unwired: 1 out]
            n3251 = Build Array(w4239, w4238) -> (w4240:string[])
            n3252 = local read "S 95"() -> (w4250:string)
            n3253 = local read "S 94"() -> (w4251:string)
            n3254 = local read "bs"() -> (w4266:string)
            n3255 = local read "as"() -> (w4267:string)
            n3256 = property on="Humidity" class="Bool (strict)"("Strings [4]"=w4240) -> ()  [unwired: 2 in, 2 out]
            n3257 = Concatenate Strings(w4266, "\r", w4267) -> ()  [unwired: 1 out]
            n3258 = property on="Rh After" class="DigNum (strict)"("Caption.Size to Text?"=TRUE ("Caption.Size to Text")) -> ()  [unwired: 2 in, 2 out]
            n3259 = local read "S 48"() -> (w4290:string)
            n3260 = local read "S 50"() -> (w4288:string)
            n3261 = local read "S 51"() -> (w4287:string)
            n3262 = local read "S 49"() -> (w4289:string)
            n3263 = local read "S 52"() -> (w4286:string)
            n3264 = local read "as"() -> (w4271:string)
            n3265 = local read "bs"() -> (w4272:string)
            n3266 = local read "S 56"() -> (w4285:string)
            n3267 = local read "S 57"() -> (w4284:string)
            n3268 = local read "S 58"() -> (w4283:string)
            n3269 = local read "S 59"() -> (w4282:string)
            n3270 = property on="OPEN" class="Bool (strict)"("Boolean Text.Text"=w4286) -> ()  [unwired: 2 in, 2 out]
            n3271 = property on="OPEN 1" class="Bool (strict)"("Boolean Text.Text"=w4290) -> ()  [unwired: 2 in, 2 out]
            n3272 = property on="OPEN 2" class="Bool (strict)"("Boolean Text.Text"=w4289) -> ()  [unwired: 2 in, 2 out]
            n3273 = property on="OPEN 3" class="Bool (strict)"("Boolean Text.Text"=w4288) -> ()  [unwired: 2 in, 2 out]
            n3274 = property on="OPEN 4" class="Bool (strict)"("Boolean Text.Text"=w4287) -> ()  [unwired: 2 in, 2 out]
            n3275 = Concatenate Strings(w4272, "\r", w4271) -> ()  [unwired: 1 out]
            n3276 = local read "S 102"() -> (w4245:string)
            n3277 = property on="КОФ1" class="DigNum (strict)"("Caption.Text"=w4285) -> ()  [unwired: 2 in, 2 out]
            n3278 = local read "S 98"() -> (w4249:string)
            n3279 = local read "S 99"() -> (w4248:string)
            n3280 = local read "S 100"() -> (w4247:string)
            n3281 = local read "S 101"() -> (w4246:string)
            n3282 = property on="КОФ2" class="DigNum (strict)"("Caption.Text"=w4284) -> ()  [unwired: 2 in, 2 out]
            n3283 = property on="КОФ3" class="DigNum (strict)"("Caption.Text"=w4283) -> ()  [unwired: 2 in, 2 out]
            n3284 = property on="КОФ4" class="DigNum (strict)"("Caption.Text"=w4282) -> ()  [unwired: 2 in, 2 out]
            n3285 = local read "bs"() -> (w4270:string)
            n3286 = local read "as"() -> (w4269:string)
            n3287 = local read "S 60"() -> (w4281:string)
            n3288 = local read "S 54"() -> (w4291:string)
            n3289 = Concatenate Strings(w4270, "\r", w4269) -> ()  [unwired: 1 out]
            n3290 = Concatenate Strings(w4291, w4281) -> ()  [unwired: 1 out]
            n3291 = local read "S 77"() -> (→"String 43":string)
            n3292 = local read "S 76"() -> (w4264:string)
            n3293 = local read "S 78"() -> (w4263:string)
            n3294 = local read "S 71"() -> (w4275:string)
            n3295 = local read "S 66"() -> (w4280:string)
            n3296 = local read "S 67"() -> (w4279:string)
            n3297 = local read "S 68"() -> (w4278:string)
            n3298 = local read "S 69"() -> (w4277:string)
            n3299 = local read "S 70"() -> (w4276:string)
            n3300 = property on="AIR TEMP" class="DigNum (strict)"("Caption.Text"=w4263) -> ()  [unwired: 2 in, 2 out]
            n3301 = property on="Set Strk" class="DigNum (strict)"("Caption.Text"=w4264) -> ()  [unwired: 2 in, 2 out]
            n3302 = property on="SPEED OUT:" class="DigNum (strict)"("Caption.Text"=w4278) -> ()  [unwired: 2 in, 2 out]
            n3303 = property on="EDIT" class="Bool (strict)"("Boolean Text.Text"=w4275) -> ()  [unwired: 2 in, 2 out]
            n3304 = local read "S 79"() -> (w4262:string)
          }
          frame #2 {
          }
        }
        n3305 = local write "Lan flag"(10.0 ("Lan flag")) -> ()
      }
      frame Enabled {
      }
    }
    n3306 = Wait (ms)(milliseconds to wait=u32 2000) -> ()  [unwired: 1 out]
    n3307 = local read "Quit"() -> (w4065:bool)
  }
  n3308 = while {
    shift-right: [w4297] -> _
    shift-left: _ -> [w4298]
    shift-right: [w4295] -> _
    shift-left: T18 {"Read Heave and Surge"="", "Bytes at Heave Port"=0.0, "Heave and Surge COM Port:"="COM9", "Com Port 2"="COM7", "Residual Due"="", "Heave COM Status 2"=TRUE, "Heave COM Status"=TRUE, "Port 2"=TRUE, "Sway PPR"=6400.0, "Surge PPR"=6400.0, "Heave PPR"=6400.0, "Sway Pitch"=2.0, "Surge Pitch"=3.0, "Heave Pitch"=4.0, "Sway Pulses/mm"=320.0, "Surge Pulses/mm"=1600.0, "Heave Pulses/mm"=1600.0, "inner loop"=0.0, "Read Heave and Surge 2"="", "String 36"="", "Write S"=FALSE, "WriteCC1"=[""], "Heave COM Loop"=0, "LastCom"="", "EXIT"=FALSE, "Error Heave"={"status"=TRUE, "code"=-1073807343, "source"=""}} -> [w4294]
    shift-right: [w4292] -> _
    shift-left: enum16{"init", "MAIN", "Panel Close"}."init" -> [w4293]
    stop <- w4296 stop-if-true
    # "HUMIDITY LOOP LOGIC"
    n3309 = case shown="\"MAIN\"" w4293 {
      tunnel: w4298 -> [w4312 w4331 w4386 w4388]
      tunnel: [w4307 w4335 w4386 w4388] -> w4297
      tunnel: [_ _ TRUE _] -> w4296
      tunnel: [w4304 w4333 w4384 w4387] -> w4295
      tunnel: w4294 -> [w4309 w4330 w4384 w4387]
      tunnel: [enum16{"init", "MAIN", "Panel Close"}."MAIN" w4325 _ _] -> w4292
      frame "init" {
        n3310 = local read "C3 :"() -> (w4299:refnum<visa-resource-name>)
        n3311 = Bundle By Name(cluster=w4309, "Heave and Surge COM Port:"=w4299) -> (w4308:T18)
        n3312 = call "Instrument fgv uno.vi"("Enum"=T32."INIT", "error in (no error) 2"=w4312, "INPUT"=w4308) -> ("error"=w4310:errorcluster, "output"=w4306:T18)  [unwired: 6 in, 1 out]
        n3313 = case shown="Error" w4310 {
          selector: w4310 -> [w4314 _]
          tunnel: [w4314 w4318] -> w4307
          tunnel: w4306 -> [w4313 w4316]
          tunnel: [w4313 w4315] -> w4305
          frame No Error {
          }
          frame Error {
            n3314 = call "Instrument fgv uno.vi"("Enum"=T32."ERROR INIT", "INPUT"=w4316) -> ("error"=w4319:errorcluster, "output"=w4315:T18)  [unwired: 7 in, 1 out]
            n3315 = call <vilib>:"Clear Errors.vi"("error in (no error)"=w4319) -> ("error out"=w4318:errorcluster)  [unwired: 5 in, 1 out]
          }
        }
        n3316 = local read "LastCom Humidity"() -> (w4302:string)
        n3317 = Unbundle By Name(w4305) -> ("Heave COM Status 2"=→"COM Status":bool, "Error Heave"=→"Error":errorcluster)  [unwired: 1 out]
        n3318 = Bundle By Name(cluster=w4305, "LastCom"=w4302) -> (w4304:T18)
      }
      frame "MAIN" {
        n3319 = Unbundle By Name(w4330) -> ("Com Port 2"=w4320:refnum<visa-resource-name>)
        n3320 = local read "C3 :"() -> (w4321:refnum<visa-resource-name>)
        n3321 = local write "COM Port Humidity :"(w4320) -> ()
        n3322 = Bundle By Name(cluster=w4330, "Heave and Surge COM Port:"=w4321) -> (w4329:T18)
        n3323 = Equal?(x=w4320, y=w4321) -> (x = y?=w4336:bool)
        n3324 = case shown="True" w4336 {
          tunnel: [w4340 w4357] -> w4335
          tunnel: w4331 -> [w4341 w4363]
          tunnel: w4329 -> [w4339 w4361]
          tunnel: [w4338 w4356] -> w4333
          frame False {
            n3325 = call <vilib>:"Clear Errors.vi"("error in (no error)"=w4341) -> ("error out"=w4337:errorcluster)  [unwired: 5 in, 1 out]
            n3326 = call "Instrument fgv uno.vi"("Enum"=T32."ERROR INIT", "error in (no error) 2"=w4337, "INPUT"=w4339) -> ("error"=w4343:errorcluster, "output"=w4338:T18)  [unwired: 6 in, 1 out]
            n3327 = call <vilib>:"Clear Errors.vi"("error in (no error)"=w4343) -> ("error out"=w4340:errorcluster)  [unwired: 5 in, 1 out]
          }
          frame True {
            n3328 = call "Instrument fgv uno.vi"("Enum"=T32."READ", "error in (no error) 2"=w4363, "INPUT"=w4361) -> ("error"=w4362:errorcluster, "output"=w4355:T18)  [unwired: 6 in, 1 out]
            n3329 = Bundle By Name(cluster=w4355, "String 36"="WRITE HUMIDITY") -> (w4354:T18)
            n3330 = case shown="True" "Write Humidity" {
              selector: "Write Humidity" -> [_ w4383]
              tunnel: w4362 -> [w4376 w4382]
              tunnel: [w4376 w4381] -> w4352
              tunnel: w4354 -> [w4375 w4379]
              tunnel: [w4375 w4378] -> w4351
              frame False {
              }
              frame True {
                n3331 = Not(x=w4383) -> (.not. x?=w4377:bool)
                n3332 = local write "Write Humidity"(w4377) -> ()
                n3333 = call "Instrument fgv uno.vi"("Enum"=T32."MANUAL WRITE", "error in (no error) 2"=w4382, "INPUT"=w4379) -> ("error"=w4381:errorcluster, "output"=w4378:T18)  [unwired: 6 in, 1 out]
              }
            }
            n3334 = Array Size(array="WriteHumidity") -> (size(s)=w4349:i32)
            n3335 = Greater Than 0?(x=w4349) -> (x > 0?=w4348:bool)
            n3336 = call "Instrument fgv uno.vi"("Enum"=T32."WRITE", "error in (no error) 2"=w4352, "WriteCC1"="WriteHumidity", "INPUT"=w4351) -> ("error"=w4359:errorcluster, "WriteCC1 2"=w4350:string[], "output"=w4358:T18)  [unwired: 5 in]
            n3337 = case shown="True" w4348 {
              tunnel: w4350 -> [_ w4365]
              frame False {
              }
              frame True {
                n3338 = local write "WriteHumidity"(w4365) -> ()
              }
            }
            n3339 = case shown="No Error" w4359 {
              selector: w4359 -> [w4366 w4369]
              tunnel: w4358 -> [w4367 w4374]
              tunnel: [w4367 w4373] -> w4356
              tunnel: [w4366 w4371] -> w4357
              frame No Error {
              }
              frame Error {
                n3340 = call <vilib>:"Clear Errors.vi"("error in (no error)"=w4369) -> ("error out"=w4368:errorcluster)  [unwired: 5 in, 1 out]
                n3341 = call "Instrument fgv uno.vi"("Enum"=T32."ERROR INIT", "error in (no error) 2"=w4368, "INPUT"=w4374) -> ("error"=w4372:errorcluster, "output"=w4373:T18)  [unwired: 6 in, 1 out]
                n3342 = call <vilib>:"Clear Errors.vi"("error in (no error)"=w4372) -> ("error out"=w4371:errorcluster)  [unwired: 5 in, 1 out]
              }
            }
            n3343 = Unbundle By Name(w4356) -> ("LastCom"=→"LastCom Humidity":string, "Read Heave and Surge"=→"Read HUMIDITY":string)
          }
        }
        n3344 = Unbundle By Name(w4333) -> ("Heave COM Status 2"=w4334:bool, "Error Heave"=w4322:errorcluster, "Bytes at Heave Port"=→"Bytes at Humidity Port  2":dbl)  [unwired: 1 out]
        n3345 = Unbundle By Name(w4322) -> ("status"=→"Humidity Port":bool)
        n3346 = Not(x=w4334) -> (.not. x?=w4323:bool)
        n3347 = local write "Error"(w4322) -> ()
        n3348 = local read "Quit"() -> (w4326:bool)
        n3349 = local write "COM Status"(w4323) -> ()
        n3350 = Select(t=enum16{"init", "MAIN", "Panel Close"}."Panel Close", s=w4326, f=enum16{"init", "MAIN", "Panel Close"}."MAIN") -> (s? t:f=w4325:enum16{"init", "MAIN", "Panel Close"})
      }
      frame "Panel Close" {
      }
      frame Default {
      }
    }
  }
  n3351 = while {
    stop <- w4390 stop-if-true
    n3352 = call <vilib>:"High Resolution Polling Wait.vi"("seconds to wait"=0.05) -> ()  [unwired: 10 in, 1 out]
    n3353 = disable-structure shown="Enabled" {
      frame Disabled {
        n3354 = local read "Read HUMIDITY"() -> (w4391:string)
        n3355 = Spreadsheet String To Array(delimiter (Tab)=",", format string="", spreadsheet string=w4391, array type (2D Dbl)=string[] []) -> (array=w4410:string[])
        n3356 = for {
          tunnel: w4410 -> [w4419] mode=indexing
          tunnel: string[] ["STATE;", "SET;", "RH;", "T;", "AMB_RH;", "AMB_T;", "PUMP;", "FAN_IN;", "FAN_OUT;", "DEHUM;", "CURRENT;", "STALL;"] -> [w4418] mode=indexing
          tunnel: [w4417] -> w4409 mode=indexing
          n3357 = Match Pattern(string=w4419, regular expression=w4418) -> (after substring=w4417:string)  [unwired: 1 in, 3 out]
        }
        n3358 = Index Array(array=w4409) -> (element #1=→"STATE :":string, element #2=→"SET :":string, element #3=w4399:string, element #4=→"T :":string, element #5=w4397:string, element #6=→"AMB_T :":string, element #7=→"PUMP :":string, element #8=→"FAN_IN :":string, element #9=→"FAN_OUT :":string, element #10=→"DEHUM :":string, element #11=→"CURRENT :":string, element #12=→"STALL :":string)  [unwired: 12 in]
        "RH :" <- w4399
        "AMB_RH :" <- w4397
        n3359 = Fract/Exp String To Number(string=w4399) -> (number=w4392:dbl)  [unwired: 3 in, 1 out]
        n3360 = Fract/Exp String To Number(string=w4397) -> (number=w4396:dbl)  [unwired: 3 in, 1 out]
        n3361 = local write "Ambient Humidity :"(w4396) -> ()
